vi "Get Test Case Classes.vi"(8 "error in (no error)":errorcluster, 11 "New Class Dialog In":refnum<class "New Class Dialog.lvclass">) -> (0 "error out":errorcluster, 3 "New Class Dialog Out":refnum<class "New Class Dialog.lvclass">)   [LabVIEW 2020, in "Process Generation.lvlib" / "New Class Dialog.lvclass"]
uses:
  New Class Dialog.lvclass
  Framework Test/Process Test/Process Test.lvclass
  C:/Users/anton/Documents/GitHub/Triarc-Framework/source/Framework Test/Base Class Test/Base Test.lvclass
  C:/Program Files (x86)/National Instruments/LabVIEW 2020/vi.lib/Asteme/LUnit/Test Case.lvclass
  C:/Users/anton/Documents/GitHub/Triarc-Framework/source/Framework Test/Process Test/Process Test.lvclass
  Framework Test/View Test/View Test.lvclass
  Framework Test/Application Test/Application Test.lvclass
  C:/Users/anton/Documents/GitHub/Triarc-Framework/source/Framework Test/Application Test/Application Test.lvclass
  C:/Users/anton/Documents/GitHub/Triarc-Framework/source/Framework Test/View Test/View Test.lvclass
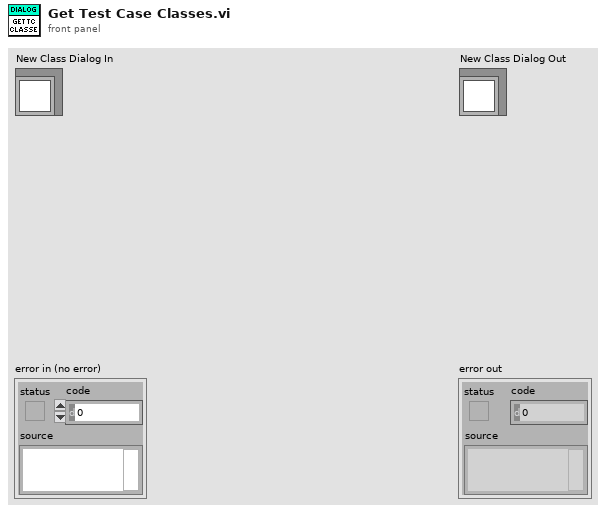
[diagram p1: front panel]
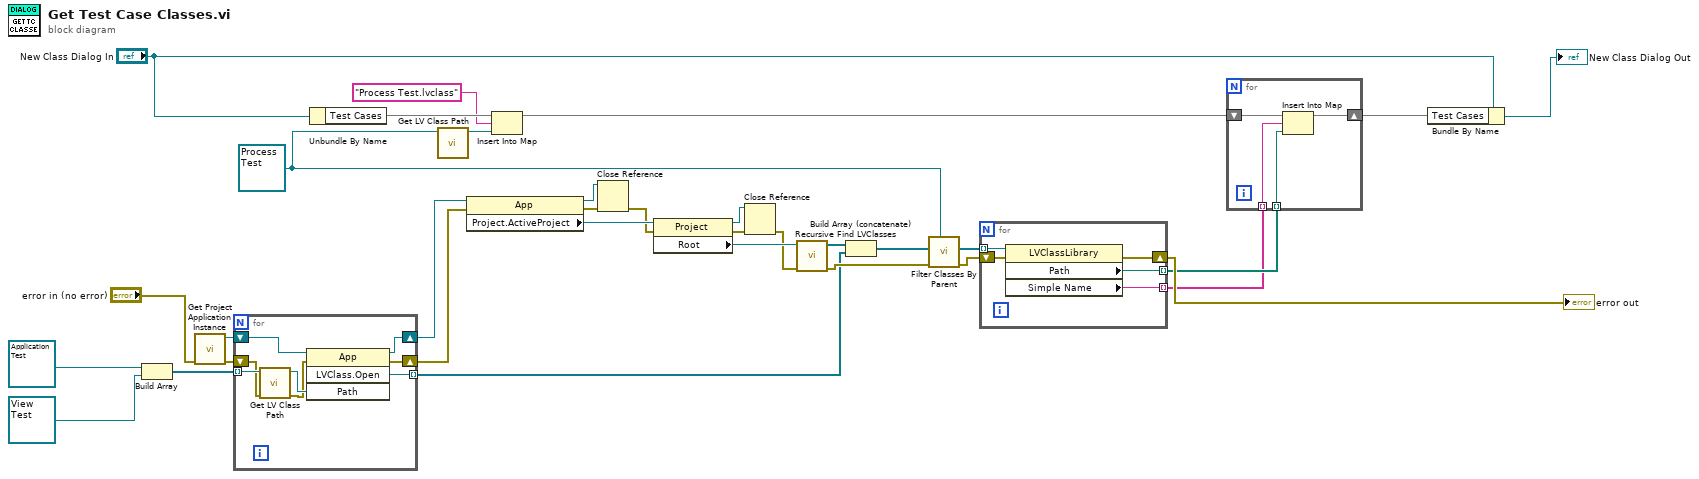
[diagram p0: block diagram]
diagram:
  w3 = refnum<class "Process Test.lvclass"> refnum ("Process Test.lvclass")
  n1 = Build Array(refnum<class "Application Test.lvclass"> refnum ("Application Test.lvclass"), refnum<class "View Test.lvclass"> refnum ("View Test.lvclass")) -> (w22:refnum<class "Process Test.lvclass">[])
  n2 = call "Get Project Application Instance.vi"("error in (no error)"="error in (no error)") -> ("error out"=w19:errorcluster, "Application out"=w18:refnum<vi>)  [unwired: 9 in]
  n3 = for {
    tunnel: w22 -> [w41] mode=indexing
    tunnel: [w39] -> w20 mode=indexing
    shift-right: [w37] -> w15
    shift-left: w18 -> [w36]
    shift-right: [w35] -> w16
    shift-left: w19 -> [w34]
    n4 = call <vilib>:"Get LV Class Path.vi"("error in (no error)"=w34, "object"=w41) -> ("error out"=w38:errorcluster, "class path"=w40:path)  [unwired: 8 in]
    n5 = invoke class="App" method="LVClass.Open"(reference=w36, error in=w38, "Path"=w40) -> (reference out=w37:refnum<vi>, error out=w35:errorcluster, "LVClass.Open"=w39:refnum<vi>)  [unwired: 1 in, 1 out]
  }
  n6 = Unbundle By Name("New Class Dialog In") -> ("Test Cases"=w33:map{string, path})
  n7 = call <vilib>:"Get LV Class Path.vi"("object"=w3) -> ("class path"=w13:path)  [unwired: 9 in, 1 out]
  n8 = property class="App"(reference=w15, error in=w16) -> (reference out=w23:refnum<vi>, error out=w25:errorcluster, "Project.ActiveProject"=w26:refnum<vi>)
  n9 = Insert Into Map(map in=w33, key="Process Test.lvclass", value=w13) -> (map out=w9:map{string, path})  [unwired: 2 out]
  n10 = Close Reference(reference=w23, error in (no error)=w25) -> (error out=w24:errorcluster)
  n11 = property class="Project"(reference=w26, error in=w24) -> (reference out=w32:refnum<vi>, error out=w31:errorcluster, "Root"=w30:refnum<vi>)
  n12 = Close Reference(reference=w32, error in (no error)=w31) -> (error out=w29:errorcluster)
  n13 = call "Recursive Find LVClasses.vi"("error in (no error)"=w29, "reference"=w30) -> ("error out"=w28:errorcluster, "Class References"=w27:refnum<vi>[])  [unwired: 8 in]
  n14 = Build Array (concatenate)(w27, w20) -> (w21:refnum<vi>[])
  n15 = call "Filter Classes By Parent.vi"("Parent Class"=w3, "error in (no error)"=w28, "Class References"=w21) -> ("error out"=w12:errorcluster, "Class References"=w10:refnum<vi>[])  [unwired: 7 in]
  n16 = for {
    tunnel: w10 -> [w46] mode=indexing
    shift-right: [w42] -> w11
    shift-left: w12 -> [w45]
    tunnel: [w44] -> w7 mode=indexing
    tunnel: [w43] -> w8 mode=indexing
    n17 = property class="LVClassLibrary"(reference=w46, error in=w45) -> (error out=w42:errorcluster, "Path"=w43:path, "Simple Name"=w44:string)  [unwired: 1 out]
  }
  "error out" <- w11
  n18 = for {
    shift-right: [w49] -> w5
    shift-left: w9 -> [w50]
    tunnel: w8 -> [w48] mode=indexing
    tunnel: w7 -> [w47] mode=indexing
    n19 = Insert Into Map(map in=w50, key=w47, value=w48) -> (map out=w49:map{string, path})  [unwired: 2 out]
  }
  n20 = Bundle By Name(cluster="New Class Dialog In", "Test Cases"=w5) -> (→"New Class Dialog Out":refnum<class "New Class Dialog.lvclass">)
